vi "0_Power_Transmission_Line_Fault_Classification(Dataset_Generation).vi"() -> ()   [LabVIEW 2020]
panel:
  in  "Test Dataset size (Per Class)":dbl=1500.0
  in  "Train Dataset size (Per Class)":dbl=5000.0
  in  "Test Dataset Folder Path":path=path "D:/Ngene/GitHub/deepltk_examples/2_Waveform_Processing/23_Power_Transmission_Line_Fault_Classification/Dataset/Test"
  in  "Train Dataset Folder Path":path=path "D:/Ngene/GitHub/deepltk_examples/2_Waveform_Processing/23_Power_Transmission_Line_Fault_Classification/Dataset/Train"
  # "This VI generates synthetic test and train datasets.\n\nInstructions:\n1. Define the sizes for the training and testing datasets for each class.\n2. Specify the location where the synthetic dataset should be stored.\n3. Execute the VI.\n4. Navigate to the  paths to observe the generated datasets."
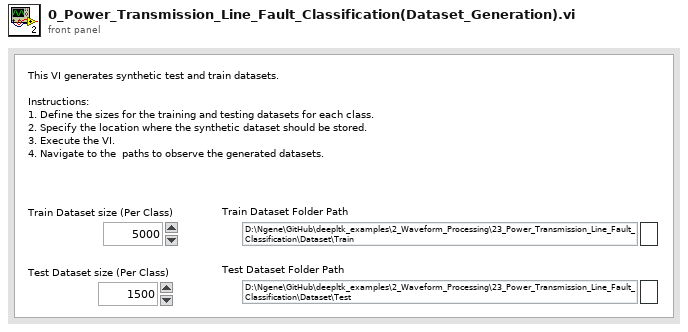
[diagram p1: front panel]
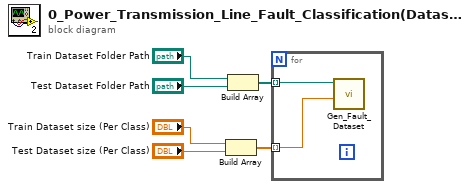
[diagram p0: block diagram]
diagram:
  n1 = Build Array("Train Dataset size (Per Class)", "Test Dataset size (Per Class)") -> (w2:dbl[])
  n2 = Build Array("Train Dataset Folder Path", "Test Dataset Folder Path") -> (w4:path[])
  n3 = for {
    tunnel: w4 -> [w8] mode=indexing
    tunnel: w2 -> [w7] mode=indexing
    n4 = call "Gen_Fault_Dataset.vi"("Number of Samples Per Class"=w7, "Dataset Folder Path"=w8) -> ()  [unwired: 9 in, 1 out]
  }
